vi "SpeakerAdjustmentLog.vi"(5 "SensorSens":dbl, 7 "RunNo.":i32, 8 "error in (no error)":errorcluster, 11 "Input cluster":T1) -> (0 "error IO":errorcluster)   [LabVIEW 2018]
uses:
  AdjustSpeakerLogCluster.ctl
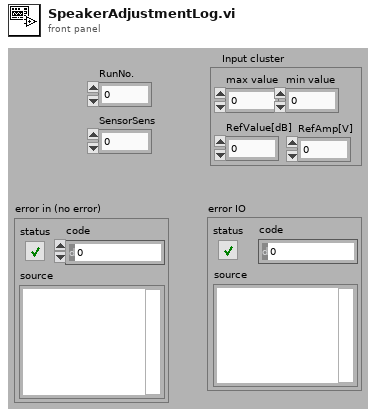
[diagram p1: front panel]
types:
  T1 = typedef "AdjustSpeakerLogCluster.ctl" = cluster{"max value":dbl, "min value":dbl, "RefValue[dB]":dbl, "RefAmp[V]":dbl}
  T2 = enum16{"open", "replace", "create", "open or create", "replace or create", "replace or create with confirmation"}
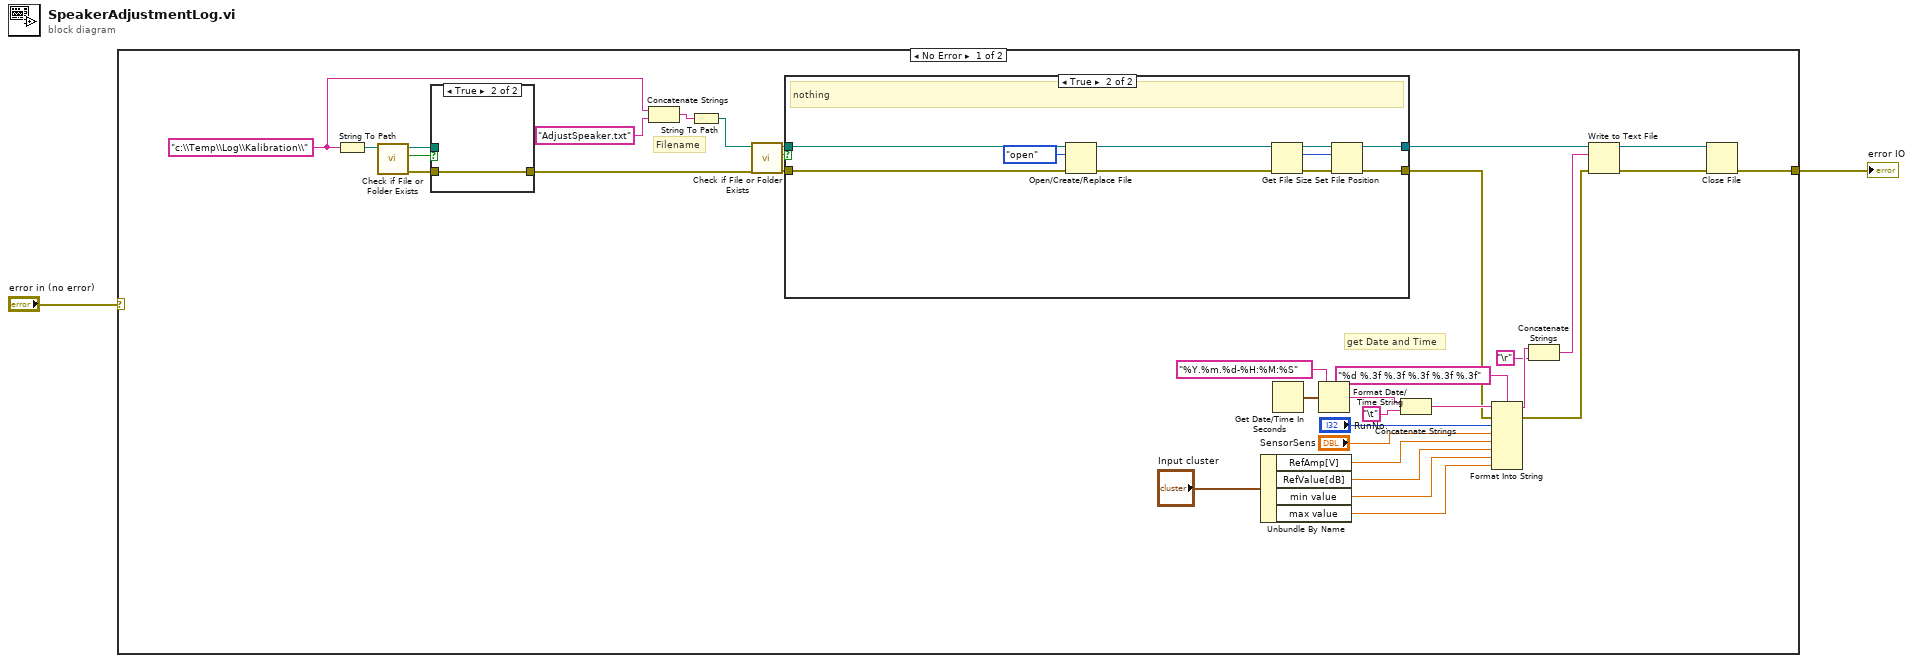
[diagram p0: block diagram]
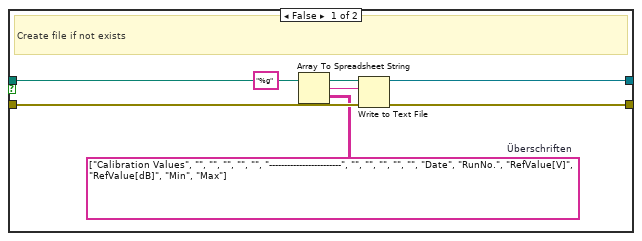
[diagram p2: hidden frame]
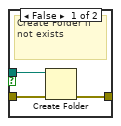
[diagram p3: hidden frame]
diagram:
  n1 = case shown="No Error" "error in (no error)" {
    selector: "error in (no error)" -> [_ w58]
    tunnel: [w23 w58] -> w2
    frame No Error {
      w28 = "c:\\Temp\\Log\\Kalibration\\" ("string")
      # "Filename"
      # "get Date and Time"
      n2 = String To Path(string=w28) -> (path=w31:path)
      n3 = call <vilib>:"Check if File or Folder Exists.vi"("path"=w31) -> ("error out"=w34:errorcluster, "file or folder exists?"=w33:bool, "dup path"=w32:path)  [unwired: 8 in]
      n4 = case shown="True" w33 {
        tunnel: w34 -> [w56 w57]
        tunnel: [w55 w57] -> w20
        tunnel: w32 -> [w54 _]
        frame False {
          # "Create Folder if not exists"
          n5 = Create Folder(path (use dialog)=w54, error in=w56) -> (error out=w55:errorcluster)  [unwired: 1 in, 2 out]
        }
        frame True {
        }
      }
      n6 = Concatenate Strings(w28, "AdjustSpeaker.txt" ("string")) -> (w30:string)
      n7 = String To Path(string=w30) -> (path=w29:path)
      n8 = call <vilib>:"Check if File or Folder Exists.vi"("error in (no error)"=w20, "path"=w29) -> ("error out"=w27:errorcluster, "file or folder exists?"=w25:bool, "dup path"=w26:path)  [unwired: 7 in]
      n9 = case shown="True" w25 {
        tunnel: [w38 w45] -> w10
        tunnel: w27 -> [w43 w52]
        tunnel: w26 -> [w42 w53]
        tunnel: [w37 w46] -> w9
        frame False {
          w41 = string[][] [["Calibration Values", "", "", "", "", ""], ["------------------------", "", "", "", "", ""], ["Date", "RunNo.", "RefValue[V]", "RefValue[dB]", "Min", "Max"]]  # Überschriften
          # "Create file if not exists"
          n10 = Array To Spreadsheet String(array=w41, 3:"%g" ("Format-String")) -> (spreadsheet string=w39:string)  [unwired: 1 in]
          n11 = Write to Text File(file (use dialog)=w42, text=w39, error in=w43) -> (refnum out=w37:refnum<file>, error out=w38:errorcluster)  [unwired: 1 in, 1 out]
        }
        frame True {
          # "nothing"
          n12 = Open/Create/Replace File(file path (use dialog)=w53, error in=w52, operation (0:open)=T2."open") -> (refnum out=w50:refnum<file>, error out=w49:errorcluster)  [unwired: 3 in, 1 out]
          n13 = Get File Size(file=w50, error in=w49) -> (refnum out=w48:refnum<file>, size (in bytes)=w44:i64, 0:w47:errorcluster)
          n14 = Set File Position(offset (in bytes) (0)=w44, refnum=w48, error in=w47) -> (refnum out=w46:refnum<file>, error out=w45:errorcluster)  [unwired: 1 in]
        }
      }
      n15 = Unbundle By Name("Input cluster") -> ("RefAmp[V]"=w6:dbl, "RefValue[dB]"=w5:dbl, "min value"=w4:dbl, "max value"=w3:dbl)
      n16 = Get Date/Time In Seconds() -> (seconds since 1Jan1904=w36:timestamp)
      n17 = Format Date/Time String(time format string (%c)="%Y.%m.%d-%H:%M:%S", seconds (now)=w36) -> (date/time string=w17:string)  [unwired: 1 in]
      n18 = Concatenate Strings(w17, "\t") -> (w14:string)
      n19 = Format Into String(format string="%d %.3f %.3f %.3f %.3f %.3f", initial string=w14, error in=w10, "RunNo.", "SensorSens", w6, w5, w4, w3) -> (resulting string=w13:string, error out=w15:errorcluster)
      n20 = Concatenate Strings(w13, "\r") -> (w12:string)
      n21 = Write to Text File(file (use dialog)=w9, text=w12, error in=w15) -> (refnum out=w22:refnum<file>, error out=w24:errorcluster)  [unwired: 1 in, 1 out]
      n22 = Close File(refnum=w22, error in=w24) -> (error out=w23:errorcluster)  [unwired: 1 out]
    }
    frame Error {
    }
  }
  "error IO" <- w2
